vi "Detect Line Change.vi"(9 "Origianl Tag":string, 10 "Original Line":T2, 11 "Final Mappings in":T1) -> (1 "Boolean":bool, 3 "Final Mappings out":T1)   [LabVIEW 2017, in "J1939 editor node.lvclass"]
uses:
  J1939 editor node.lvclass
  Mappings.ctl
  <vilib>/NI/Tag Bus Module Framework/channel/TBM channel.lvclass
  module/configuration/Line.ctl
  Map.ctl
  module/configuration/J1939 configuration.lvclass
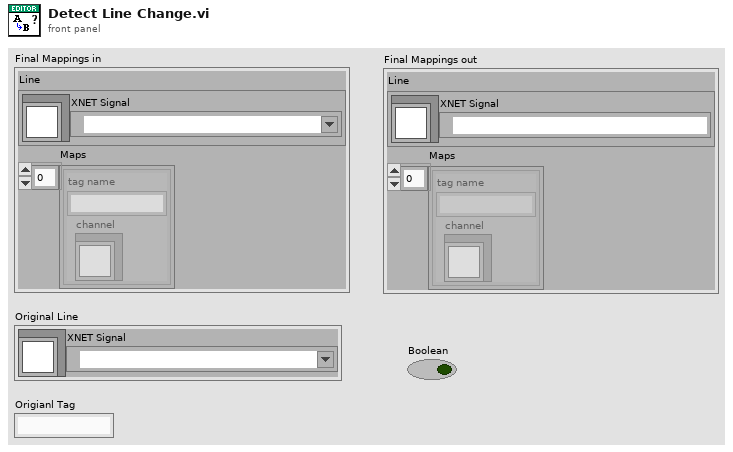
[diagram p1: front panel]
types:
  T1 = typedef "J1939 editor node.lvclass/Mappings.ctl" = cluster{"Line":T2, "Maps":T3[]}
  T2 = typedef "J1939 configuration.lvclass/Line.ctl" = cluster{"channel":refnum<class "TBM channel.lvclass">, "XNET Signal":refnum<k21>}
  T3 = typedef "J1939 editor node.lvclass/Map.ctl" = cluster{"channel":refnum<class "TBM channel.lvclass">, "tag name":string}
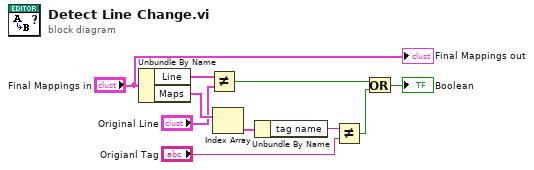
[diagram p0: block diagram]
diagram:
  n1 = Unbundle By Name("Final Mappings in") -> ("Line"=w4:T2, "Maps"=w5:T3[])
  n2 = Not Equal?(x=w4, y="Original Line") -> (x != y?=w2:bool)
  n3 = Index Array(array=w5) -> (element=w6:T3)  [unwired: 1 in]
  n4 = Unbundle By Name(w6) -> ("tag name"=w7:string)
  n5 = Not Equal?(x=w7, y="Origianl Tag") -> (x != y?=w10:bool)
  n6 = Or(x=w2, y=w10) -> (x .or. y?=→"Boolean":bool)
  "Final Mappings out" <- "Final Mappings in"
